vi "Untitled 63.vi"   [LabVIEW 2013]
uses:
  <vilib>/Analysis/Matrix/Datatypes/RealMatrix.ctl
  <vilib>/robotics/Kinematics/Analytical/Initialize Generic Serial Arm.vi
  <vilib>/robotics/Kinematics/Link/Joint Type.ctl
  <vilib>/robotics/Kinematics/Link/NI_Robotics_Link.lvclass
  <vilib>/Analysis/Matrix/NI_Matrix.lvlib
  <vilib>/robotics/Kinematics/Analytical/NI_Robotics_AnalyticKinematics.lvlib
  <vilib>/robotics/Kinematics/Robot/NI_Robotics_Serial Robot Arm.lvclass
types:
  T1 = typedef "NI_Matrix.lvlib/RealMatrix.ctl" = dbl[][]
  T2 = cluster{"mass":dbl, "gear ratio":dbl, "motor inertia":dbl, "center of gravity":dbl[], "viscous friction":dbl, "positive coulomb friction":dbl, "negative coulomb friction":dbl, "inertia matrix":T1}[]
  T3 = typedef "NI_Robotics_Link.lvclass/Joint Type.ctl" = enum16{"Revolute", "Prismatic"}
  T4 = cluster{"Twist Angle":dbl, "Length":dbl, "Rotation Angle":dbl, "Offset Distance":dbl, "Joint Type":T3, "Joint Coordinate Offset":dbl}[]
  T5 = typedef "DH Kinematic Parameters.ctl" = cluster{"twist angle":dbl, "length":dbl, "rotation angle":dbl, "offset distance":dbl, "joint type":T3, "joint coordinate offset":dbl}
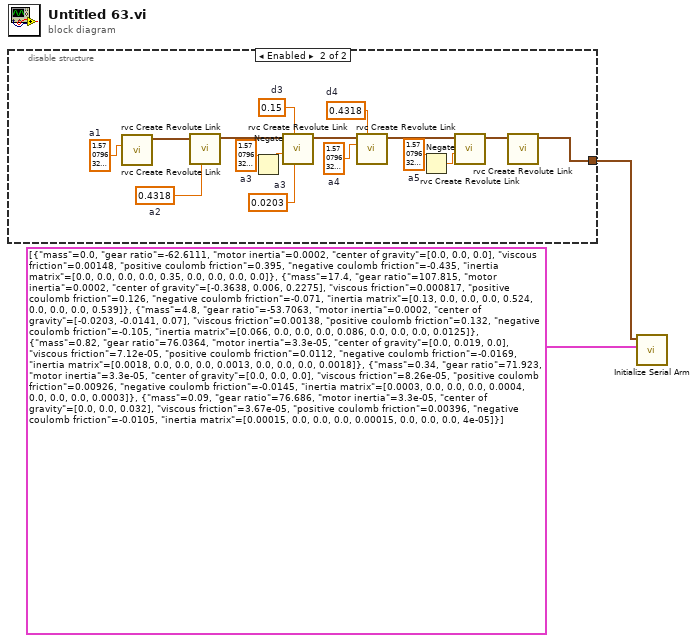
[diagram p0: block diagram]
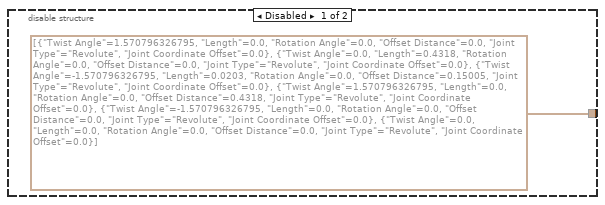
[diagram p2: hidden frame]
diagram:
  n1 = disable-structure shown="Enabled" {
    disable-tunnel: [T4 [{"Twist Angle"=1.570796326795, "Length"=0.0, "Rotation Angle"=0.0, "Offset Distance"=0.0, "Joint Type"=enum."Revolute", "Joint Coordinate Offset"=0.0}, {"Twist Angle"=0.0, "Length"=0.4318, "Rotation Angle"=0.0, "Offset Distance"=0.0, "Joint Type"=enum."Revolute", "Joint Coordinate Offset"=0.0}, {"Twist Angle"=-1.570796326795, "Length"=0.0203, "Rotation Angle"=0.0, "Offset Distance"=0.15005, "Joint Type"=enum."Revolute", "Joint Coordinate Offset"=0.0}, {"Twist Angle"=1.570796326795, "Length"=0.0, "Rotation Angle"=0.0, "Offset Distance"=0.4318, "Joint Type"=enum."Revolute", "Joint Coordinate Offset"=0.0}, {"Twist Angle"=-1.570796326795, "Length"=0.0, "Rotation Angle"=0.0, "Offset Distance"=0.0, "Joint Type"=enum."Revolute", "Joint Coordinate Offset"=0.0}, {"Twist Angle"=0.0, "Length"=0.0, "Rotation Angle"=0.0, "Offset Distance"=0.0, "Joint Type"=enum."Revolute", "Joint Coordinate Offset"=0.0}] w4] -> w2
    frame Disabled {
    }
    frame Enabled {
      w6 = 1.5707963267948966  # a5
      w7 = 0.4318  # d4
      w8 = 1.5707963267948966  # a4
      w10 = 1.5707963267948966  # a3
      w11 = 0.15  # d3
      w12 = 0.0203  # a3
      w16 = 0.4318  # a2
      w18 = 1.5707963267948966  # a1
      n2 = call "rvc Create Revolute Link.vi"("twist angle (alpha)"=w18) -> ("Array"=w17:T5[])  [unwired: 10 in]
      n3 = call "rvc Create Revolute Link.vi"("length (a)"=w16, "Array 2"=w17) -> ("Array"=w15:T5[])  [unwired: 9 in]
      n4 = Negate(x=w10) -> (-x=w9:dbl)
      n5 = call "rvc Create Revolute Link.vi"("length (a)"=w12, "offset distance (d)"=w11, "twist angle (alpha)"=w9, "Array 2"=w15) -> ("Array"=w14:T5[])  [unwired: 7 in]
      n6 = call "rvc Create Revolute Link.vi"("offset distance (d)"=w7, "twist angle (alpha)"=w8, "Array 2"=w14) -> ("Array"=w13:T5[])  [unwired: 8 in]
      n7 = Negate(x=w6) -> (-x=w5:dbl)
      n8 = call "rvc Create Revolute Link.vi"("twist angle (alpha)"=w5, "Array 2"=w13) -> ("Array"=w19:T5[])  [unwired: 9 in]
      n9 = call "rvc Create Revolute Link.vi"("Array 2"=w19) -> ("Array"=w4:T5[])  [unwired: 10 in]
    }
  }
  n10 = call-poly <vilib>:"Initialize Serial Arm.vi"("dynamic parameters"=T2 [{"mass"=0.0, "gear ratio"=-62.6111, "motor inertia"=0.0002, "center of gravity"=[0.0, 0.0, 0.0], "viscous friction"=0.00148, "positive coulomb friction"=0.395, "negative coulomb friction"=-0.435, "inertia matrix"=[[0.0, 0.0, 0.0], [0.0, 0.35, 0.0], [0.0, 0.0, 0.0]]}, {"mass"=17.4, "gear ratio"=107.815, "motor inertia"=0.0002, "center of gravity"=[-0.3638, 0.006, 0.2275], "viscous friction"=0.000817, "positive coulomb friction"=0.126, "negative coulomb friction"=-0.071, "inertia matrix"=[[0.13, 0.0, 0.0], [0.0, 0.524, 0.0], [0.0, 0.0, 0.539]]}, {"mass"=4.8, "gear ratio"=-53.7063, "motor inertia"=0.0002, "center of gravity"=[-0.0203, -0.0141, 0.07], "viscous friction"=0.00138, "positive coulomb friction"=0.132, "negative coulomb friction"=-0.105, "inertia matrix"=[[0.066, 0.0, 0.0], [0.0, 0.086, 0.0], [0.0, 0.0, 0.0125]]}, {"mass"=0.82, "gear ratio"=76.0364, "motor inertia"=3.3e-05, "center of gravity"=[0.0, 0.019, 0.0], "viscous friction"=7.12e-05, "positive coulomb friction"=0.0112, "negative coulomb friction"=-0.0169, "inertia matrix"=[[0.0018, 0.0, 0.0], [0.0, 0.0013, 0.0], [0.0, 0.0, 0.0018]]}, {"mass"=0.34, "gear ratio"=71.923, "motor inertia"=3.3e-05, "center of gravity"=[0.0, 0.0, 0.0], "viscous friction"=8.26e-05, "positive coulomb friction"=0.00926, "negative coulomb friction"=-0.0145, "inertia matrix"=[[0.0003, 0.0, 0.0], [0.0, 0.0004, 0.0], [0.0, 0.0, 0.0003]]}, {"mass"=0.09, "gear ratio"=76.686, "motor inertia"=3.3e-05, "center of gravity"=[0.0, 0.0, 0.032], "viscous friction"=3.67e-05, "positive coulomb friction"=0.00396, "negative coulomb friction"=-0.0105, "inertia matrix"=[[0.00015, 0.0, 0.0], [0.0, 0.00015, 0.0], [0.0, 0.0, 4e-05]]}] ("Array"), "kinematic parameters"=w2) -> ()  [unwired: 8 in, 2 out]
